vi "StatIntialse.vi"(0 "Init cluster 2":T1, 1 "Set Stability":T2(ring)=enum."Standard", 2 "Default\n Filter":T3(ring)=enum."10 kHz", 3 "error in (no error)":errorcluster, 4 "Default\nCurrent range":T4(ring)=enum."10 mA") -> (7 "Init cluster":T1, 10 "error out":errorcluster)   [LabVIEW 2022 SP3]
uses:
  IVIUM/IVIUM_remdriver.lvlib
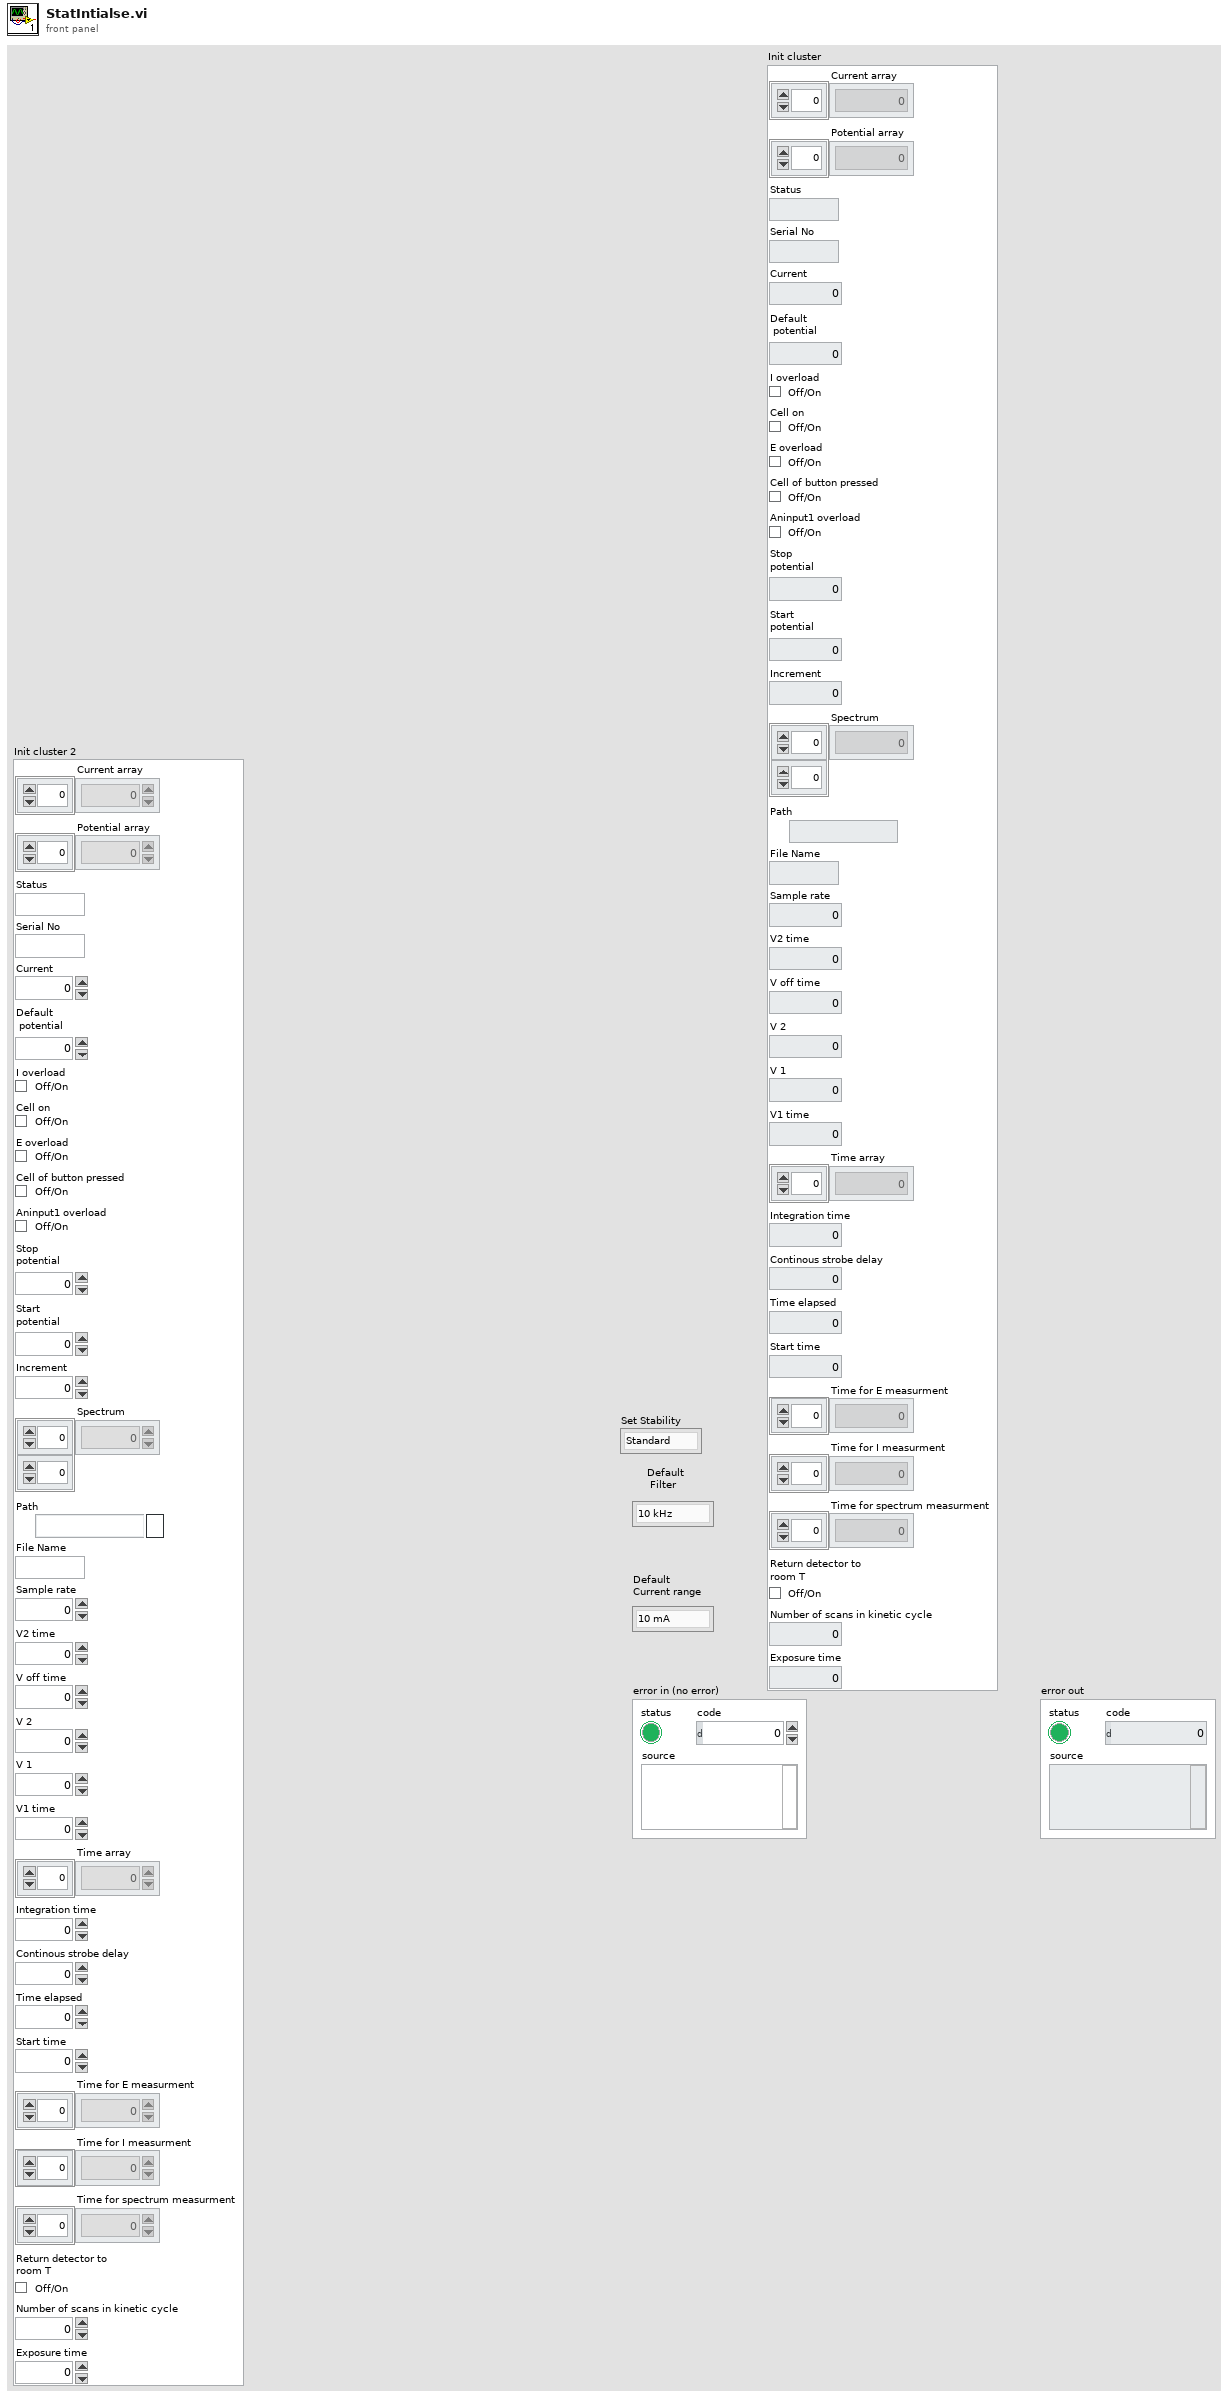
[diagram p1: front panel]
types:
  T1 = cluster{"Current array":dbl[], "Potential array":dbl[], "Status":string, "Serial No":string, "Current":dbl, "Default\n potential":dbl, "I overload":bool, "Cell on":bool, "E overload":bool, "Cell of button pressed":bool, "Aninput1 overload":bool, "Stop \npotential":dbl, "Start \npotential":dbl, "Increment":dbl, "Spectrum":dbl[][], "Path":path, "File Name":string, "Sample rate":dbl, "V2 time":dbl, "V off time":dbl, "V 2":dbl, "V 1":dbl, "V1 time":dbl, "Time array":dbl[], "Integration time":i32, "Continous strobe delay":i32, "Time elapsed ":i32, "Start time":i32, "Time for E measurment":i32[], "Time for I measurment ":i32[], "Time for spectrum measurment":i32[], "Return detector to \nroom T":bool, "Number of scans in kinetic cycle":i32, "Exposure time":i32}
  T2 = enum16{"High Speed", "Standard", "High Stability"}
  T3 = enum16{"1 MHz", "100 kHz", "10 kHz", "1 kHz", "10 Hz"}
  T4 = enum16{"10 A", "1 A", "100 mA", "10 mA", "1 mA", "100 uA", "10 uA", "1 uA", "100 nA", "10 nA", "1 nA", "100 pA", "10 pA", "1 pA"}
  T5 = enum16{"off", "EStat4EL", "EStat2EL", "EStatDummy1", "EStatDummy2", "EStatDummy3", "EStatDummy4", "IStat4EL", "IStat2EL", "IStatDummy", "BiStat4EL", "BiStat2EL"}
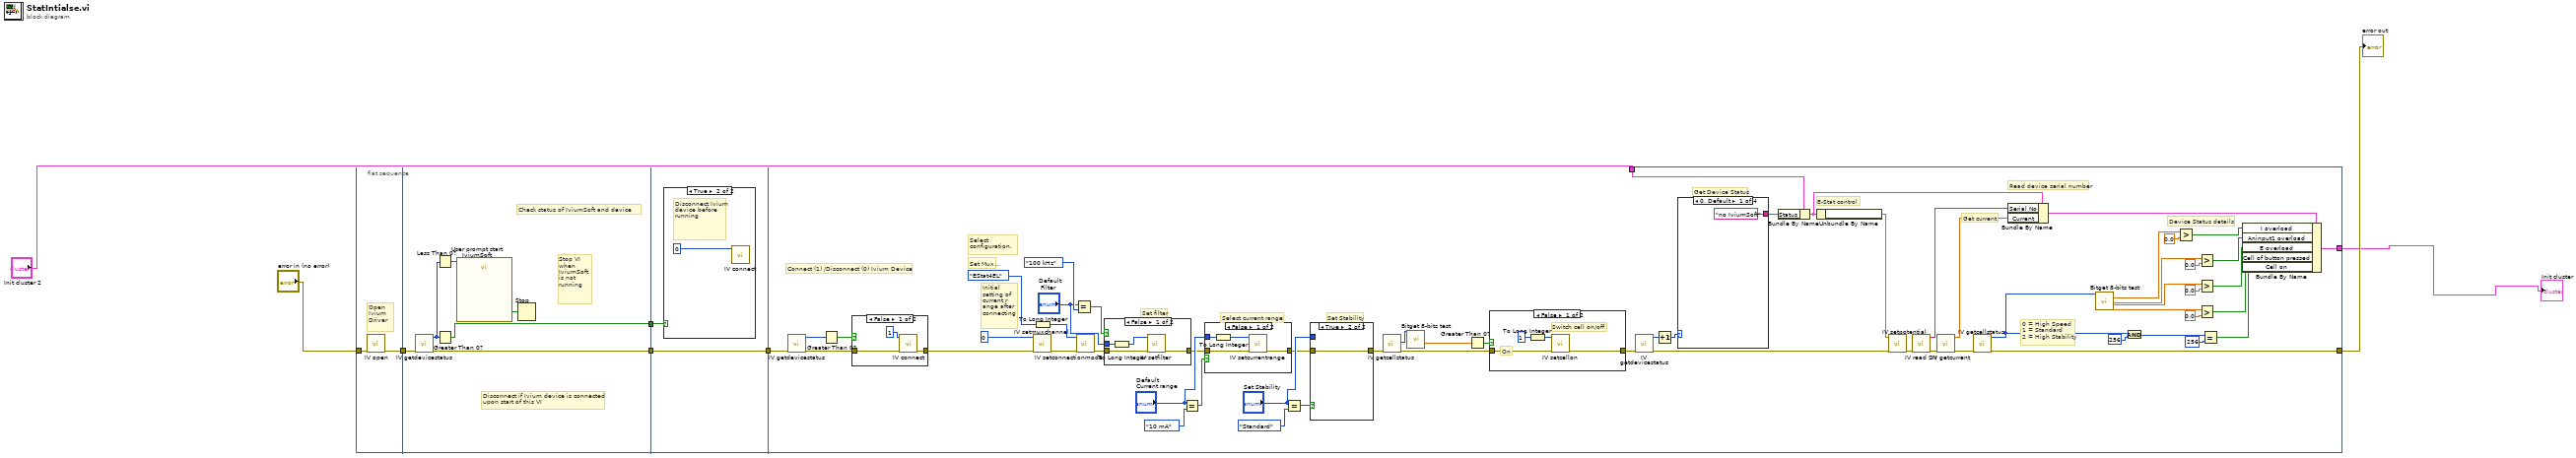
[diagram p0: block diagram]
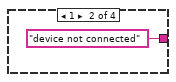
[diagram p5: hidden frame]
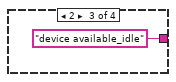
[diagram p6: hidden frame]
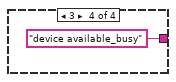
[diagram p7: hidden frame]
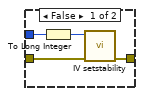
[diagram p8: hidden frame]
diagram:
  n1 = flat-sequence {
    tunnel: [w10] -> w7
    tunnel: "error in (no error)" -> [w9]
    tunnel: w7 -> [w13]
    tunnel: [w12] -> w5
    tunnel: [w11] -> w3
    tunnel: w5 -> [w18]
    tunnel: [w18] -> w4
    tunnel: w3 -> [w17]
    tunnel: "Init cluster 2" -> [w32]
    tunnel: [w43] -> w8
    tunnel: w4 -> [w23]
    tunnel: [w21] -> w1
    frame #0 {
      # "Open Ivium Driver"
      n2 = call "IV open.vi"("error in (no error)"=w9) -> ("error out"=w10:errorcluster)  [unwired: 9 in, 1 out]
    }
    frame #1 {
      # "Check status of IviumSoft and device"
      # "Stop VI when IviumSoft is not running"
      # "Disconnect if Ivium device is connected \nupon start of this VI"
      n3 = call "IV getdevicestatus.vi"("error in (no error)"=w13) -> ("error out"=w12:errorcluster, "return type"=w16:i32)  [unwired: 9 in]
      n4 = Less Than 0?(x=w16) -> (x < 0?=w14:bool)
      n5 = Greater Than 0?(x=w16) -> (x > 0?=w11:bool)
      n6 = call "User prompt start IviumSoft.vi"("Enable"=w14) -> ("OK"=w15:bool)  [unwired: 17 in, 1 out]
      n7 = Stop(stop? (T)=w15) -> ()
    }
    frame #2 {
      n8 = case shown="True" w17 {
        frame False {
        }
        frame True {
          # "Disconnect Ivium device before running"
          n9 = call "IV connect.vi"("devconnect"=0) -> ()  [unwired: 8 in, 3 out]
        }
      }
    }
    frame #3 {
      # "Device Status details"
      # "Get current"
      # "Set Mux channel"
      # "0 = High Speed\n1 = Standard \n2 = High Stability"
      # "Set Stability"
      # "Set filter"
      # "E-Stat control"
      # "Get Device Status"
      # "Select current range"
      # "Select configuration,"
      # "Read device serial number"
      # "Initial setting of current r\nange after connecting"
      # "Connect (1) /Disconnect (0) Ivium Device"
      n10 = call "IV getdevicestatus.vi"("error in (no error)"=w23) -> ("error out"=w40:errorcluster, "return type"=w42:i32)  [unwired: 9 in]
      n11 = Greater Than 0?(x=w42) -> (x > 0?=w41:bool)
      n12 = case shown="False" w41 {
        tunnel: [w81 w82] -> w20
        tunnel: w40 -> [w79 w82]
        frame False {
          n13 = call "IV connect.vi"("error in (no error)"=w79, "devconnect"=1) -> ("error out"=w81:errorcluster)  [unwired: 7 in, 2 out]
        }
        frame True {
        }
      }
      n14 = call "IV setmuxchannel.vi"("error in (no error)"=w20, "value"=0) -> ("error out"=w39:errorcluster)  [unwired: 7 in, 2 out]
      n15 = To Long Integer(number=T5."EStat4EL" ("Configuration")) -> (32bit integer=w38:i32)
      n16 = Equal?(x="Default\n Filter", y=T3."100 kHz" ("Set Filter")) -> (x = y?=w72:bool)
      n17 = call "IV setconnectionmode.vi"("error in (no error)"=w39, "value"=w38) -> ("error out"=w36:errorcluster)  [unwired: 7 in, 2 out]
      n18 = case shown="False" w72 {
        tunnel: "Default\n Filter" -> [w100 _]
        tunnel: [w98 w101] -> w37
        tunnel: w36 -> [w97 w101]
        frame False {
          n19 = To Long Integer(number=w100) -> (32bit integer=w99:i32)
          n20 = call "IV setfilter.vi"("error in (no error)"=w97, "value"=w99) -> ("error out"=w98:errorcluster)  [unwired: 7 in, 2 out]
        }
        frame True {
        }
      }
      n21 = Equal?(x="Default\nCurrent range", y=T4."10 mA") -> (x = y?=w76:bool)
      n22 = case shown="False" w76 {
        tunnel: "Default\nCurrent range" -> [w104 _]
        tunnel: [w103 w106] -> w35
        tunnel: w37 -> [w102 w106]
        frame False {
          n23 = To Long Integer(number=w104) -> (32bit integer=w105:i32)
          n24 = call "IV setcurrentrange.vi"("error in (no error)"=w102, "value"=w105) -> ("error out"=w103:errorcluster)  [unwired: 7 in, 2 out]
        }
        frame True {
        }
      }
      n25 = Equal?(x="Set Stability", y=T2."Standard" ("Set Stability")) -> (x = y?=w74:bool)
      n26 = case shown="True" w74 {
        tunnel: "Set Stability" -> [w95 _]
        tunnel: [w93 w96] -> w34
        tunnel: w35 -> [w92 w96]
        frame False {
          n27 = To Long Integer(number=w95) -> (32bit integer=w94:i32)
          n28 = call "IV setstability.vi"("error in (no error)"=w92, "value"=w94) -> ("error out"=w93:errorcluster)  [unwired: 7 in, 2 out]
        }
        frame True {
        }
      }
      n29 = call "IV getcellstatus.vi"("error in (no error)"=w34) -> ("error out"=w45:errorcluster, "return type"=w48:i32)  [unwired: 8 in, 1 out]
      n30 = call "Bitget 8-bits test.vi"("x"=w48) -> ("f"=w47:dbl)  [unwired: 19 in, 7 out]
      n31 = Greater Than 0?(x=w47) -> (x > 0?=w46:bool)
      n32 = case shown="False" w46 {
        tunnel: w45 -> [w84 w87]
        tunnel: [w83 w87] -> w33
        frame False {
          # "On"
          # "Switch cell on/off"
          n33 = To Long Integer(number=1) -> (32bit integer=w86:i32)
          n34 = call "IV setcellon.vi"("error in (no error)"=w84, "cellon"=w86) -> ("error out"=w83:errorcluster)  [unwired: 7 in, 2 out]
        }
        frame True {
          # "If the cell is already\n on do nothing here"
        }
      }
      n35 = call "IV getdevicestatus.vi"("error in (no error)"=w33) -> ("error out"=w28:errorcluster, "return type"=w69:i32)  [unwired: 9 in]
      n36 = Increment(x=w69) -> (x+1=w68:i32)
      n37 = case shown="0, Default" w68 {
        tunnel: ["no IviumSoft" "device not connected" "device available_idle" "device available_busy"] -> w54
        frame 0, Default {
        }
        frame 1 {
        }
        frame 2 {
        }
        frame 3 {
        }
      }
      n38 = Bundle By Name(cluster=w32, "Status"=w54) -> (w29:T1)
      n39 = Unbundle By Name(w29) -> ("Default\n potential"=w31:dbl)
      n40 = call "IV setpotential.vi"("error in (no error)"=w28, "value"=w31) -> ("error out"=w30:errorcluster)  [unwired: 7 in, 2 out]
      n41 = call "IV read SN.vi"("error in (no error)"=w30) -> ("error out"=w27:errorcluster, "sntext out"=w53:string)  [unwired: 8 in, 1 out]
      n42 = call "IV getcurrent.vi"("error in (no error)"=w27) -> ("error out"=w24:errorcluster, "value out"=w26:dbl)  [unwired: 8 in, 1 out]
      n43 = call "IV getcellstatus.vi"("error in (no error)"=w24) -> ("error out"=w43:errorcluster, "devcellstatus out"=w59:i32)  [unwired: 8 in, 1 out]
      n44 = Bundle By Name(cluster=w29, "Serial No"=w53, "Current"=w26) -> (w25:T1)
      n45 = call "Bitget 8-bits test.vi"("x"=w59) -> ("c"=w63:dbl, "e"=w61:dbl, "f"=w62:dbl, "h"=w60:dbl)  [unwired: 19 in, 4 out]
      n46 = And(x=w59, y=256) -> (x .and. y?=w57:i32)
      n47 = Greater?(x=w63, y=0.0) -> (0:w52:bool)
      n48 = Greater?(x=w61, y=0.0) -> (0:w51:bool)
      n49 = Greater?(x=w62, y=0.0) -> (0:w50:bool)
      n50 = Greater?(x=w60, y=0.0) -> (0:w22:bool)
      n51 = Equal?(x=w57, y=256) -> (x = y?=w49:bool)
      n52 = Bundle By Name(cluster=w25, "I overload"=w52, "Aninput1 overload"=w51, "E overload"=w50, "Cell of button pressed"=w22, "Cell on"=w49) -> (w21:T1)
    }
  }
  "error out" <- w8
  "Init cluster" <- w1
